vi "Watchdog.vi"(1 "Encoder":dbl format="%#_13g", 2 "Motor Input":dbl) -> (0 "Motor Output":dbl)   [LabVIEW 2016]
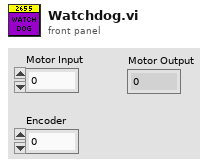
[diagram p1: front panel]
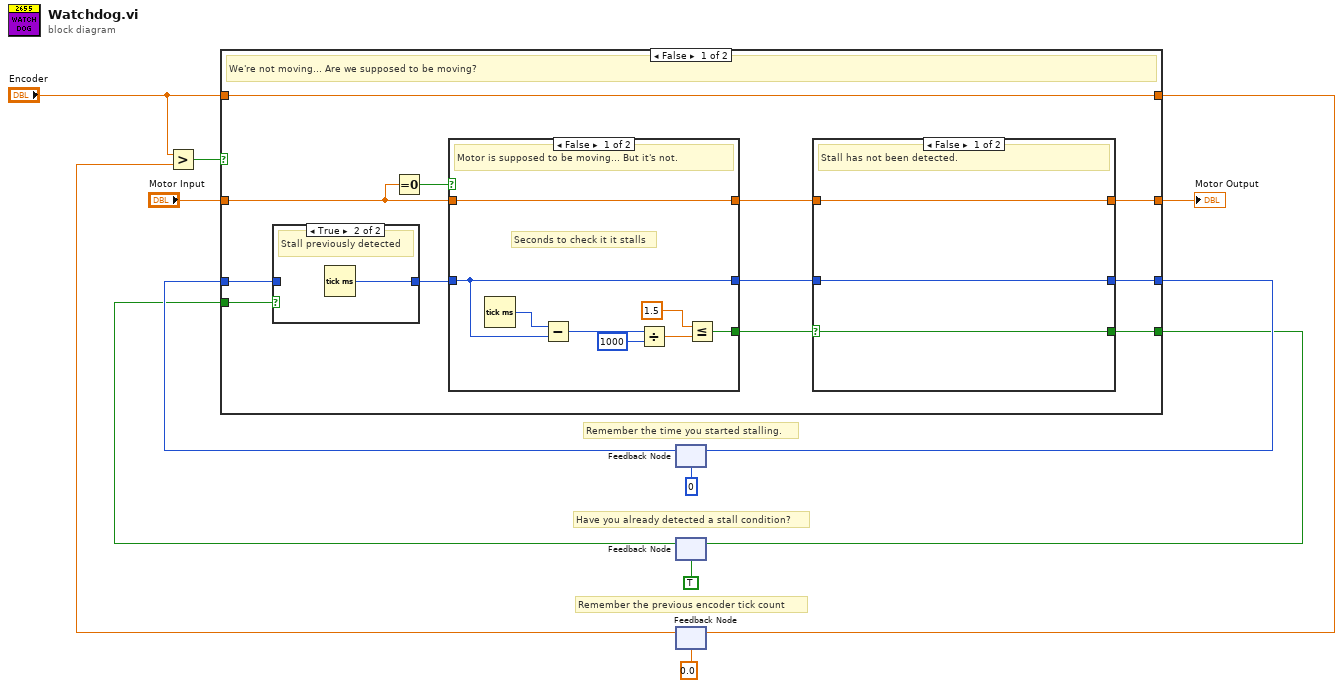
[diagram p0: block diagram]
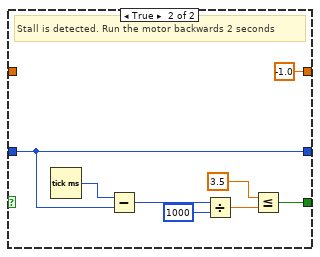
[diagram p2: hidden frame]
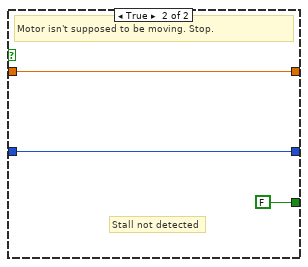
[diagram p4: hidden frame]
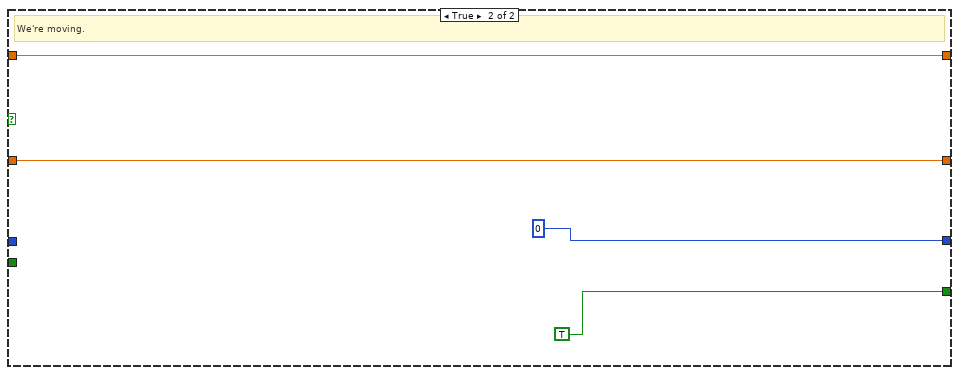
[diagram p5: hidden frame]
diagram:
  # "Remember the previous encoder tick count"
  # "Have you already detected a stall condition?"
  # "Remember the time you started stalling."
  n1 = feedback #1(u32 0 ("millisecond timer value")) -> (w13:u32)
  n2 = feedback #2(TRUE ("f")) -> (w8:bool)
  n3 = feedback #3(0.0 ("Encoder")) -> (w7:dbl)
  n4 = Greater?(x="Encoder", y=w7) -> (0:w5:bool)
  n5 = case shown="False" w5 {
    tunnel: w13 -> [w24 _]
    tunnel: [w16 0] -> w12
    tunnel: [w18 TRUE ("f")] -> w9
    tunnel: w8 -> [w22 _]
    tunnel: [w21 w51] -> w6
    tunnel: "Encoder" -> [w21 w51]
    tunnel: "Motor Input" -> [w20 w50]
    tunnel: [w14 w50] -> w3
    frame False {
      # "We're not moving... Are we supposed to be moving?"
      n6 = case shown="True" w22 {
        tunnel: [w37 w38] -> w23
        tunnel: w24 -> [w37 _]
        frame False {
          # "Stall not detected"
        }
        frame True {
          # "Stall previously detected"
          n7 = Tick Count (ms)() -> (millisecond timer value=w38:u32)
        }
      }
      n8 = Equal To 0?(x=w20) -> (x = 0?=w25:bool)
      n9 = case shown="False" w25 {
        tunnel: [w41 FALSE ("f")] -> w19
        tunnel: w23 -> [w40 w48]
        tunnel: [w40 w48] -> w17
        tunnel: [w39 w47] -> w15
        tunnel: w20 -> [w39 w47]
        frame False {
          # "Seconds to check it it stalls"
          # "Motor is supposed to be moving... But it's not."
          n10 = Tick Count (ms)() -> (millisecond timer value=w46:u32)
          n11 = Subtract(x=w46, y=w40) -> (x-y=w45:u32)
          n12 = Divide(x=w45, y=u32 1000) -> (x/y=w43:dbl)
          n13 = Less Or Equal?(x=1.5, y=w43) -> (x <= y?=w41:bool)
        }
        frame True {
          # "Stall not detected"
          # "Motor isn't supposed to be moving. Stop."
        }
      }
      n14 = case shown="False" w19 {
        selector: w19 -> [w28 _]
        tunnel: [w28 w29] -> w18
        tunnel: w17 -> [w27 w30]
        tunnel: [w27 w30] -> w16
        tunnel: w15 -> [w26 _]
        tunnel: [w26 -1.0 ("Motor Input")] -> w14
        frame False {
          # "Stall has not been detected."
        }
        frame True {
          # "Stall is detected. Run the motor backwards 2 seconds"
          n15 = Tick Count (ms)() -> (millisecond timer value=w35:u32)
          n16 = Subtract(x=w35, y=w30) -> (x-y=w34:u32)
          n17 = Divide(x=w34, y=u32 1000) -> (x/y=w32:dbl)
          n18 = Less Or Equal?(x=3.5, y=w32) -> (x <= y?=w29:bool)
        }
      }
    }
    frame True {
      # "We're moving."
    }
  }
  "Motor Output" <- w3
  n19 = feedback-in #1(w12) -> ()
  n20 = feedback-in #2(w9) -> ()
  n21 = feedback-in #3(w6) -> ()
